vi "Get Optimal Fourier Order.vi"(8 "Error In":errorcluster, 9 "[b_k]":dbl[](array[numeric]), 11 "[a_k]":dbl[](array[numeric])) -> (0 "Error Out":errorcluster, 1 "Smoothed Power Spectrum":dbl[](array[numeric]), 3 "Optimal Fourier Order":i32)   [LabVIEW 2019]
uses:
  <vilib>/addons/_Advanced Signal Processing/NI_AdvSigProcTSA.lvlib
panel:
  out "Power Spectrum":dbl[](array[numeric])
  out "Graph":dbl[][](graph)
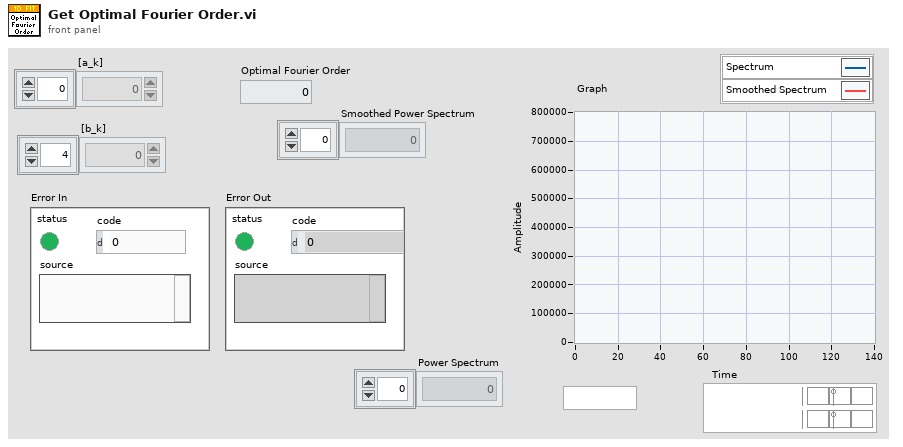
[diagram p1: front panel]
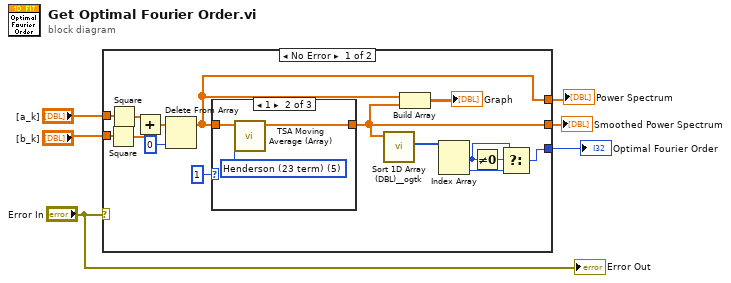
[diagram p0: block diagram]
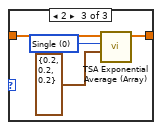
[diagram p3: hidden frame]
diagram:
  n1 = case shown="No Error" "Error In" {
    tunnel: "[a_k]" -> [w20 _]
    tunnel: "[b_k]" -> [w19 _]
    tunnel: [w12 _] -> w4
    tunnel: [w8 _] -> w3
    tunnel: [w10 _] -> w1
    frame No Error {
      n2 = Square(x=w19) -> (x^2=w18:dbl[])
      n3 = Square(x=w20) -> (x^2=w21:dbl[])
      n4 = Add(x=w21, y=w18) -> (x+y=w9:dbl[])
      n5 = Delete From Array(array=w9, index=0) -> (array with subset deleted=w8:dbl[])  [unwired: 1 in, 1 out]
      n6 = case shown="1" 1 {
        tunnel: w8 -> [w22 w25 w29]
        tunnel: [w22 w24 w28] -> w10
        frame 0, Default {
        }
        frame 1 {
          w23 = 5 items=["Spencer (15 term)"=1, "Henderson (7 term)"=2, "Henderson (9 term)"=3, "Henderson (13 term)"=4, "Henderson (23 term)"=5] ("method")
          n7 = call <vilib>:"TSA Moving Average (Array).vi"("method"=w23, "Xt"=w25) -> ("Xt out"=w24:dbl[])  [unwired: 8 in, 1 out]
        }
        frame 2 {
          w27 = u16 0 items=["Single", "Double", "Triple"] ("exponential type")
          n8 = call <vilib>:"TSA Exponential Average (Array).vi"("exponential factors"=cluster{"level":dbl, "trend":dbl, "season":dbl} {"level"=0.2, "trend"=0.2, "season"=0.2}, "exponential type"=w27, "Xt"=w29) -> ("Xt averaged"=w28:dbl[])  [unwired: 7 in, 1 out]
        }
      }
      n9 = call <userlib>:"Sort 1D Array (DBL)__ogtk.vi"("Array in"=w10) -> ("Sorted Pointers"=w16:i32[])  [unwired: 9 in, 1 out]
      n10 = Build Array(w8, w10) -> (→"Graph":dbl[][])
      n11 = Index Array(array=w16) -> (element #1=w14:i32, element #2=w13:i32)  [unwired: 2 in]
      n12 = Not Equal To 0?(x=w14) -> (x != 0?=w15:bool)
      n13 = Select(t=w14, s=w15, f=w13) -> (s? t:f=w12:i32)
    }
    frame Error {
    }
  }
  "Optimal Fourier Order" <- w4
  "Smoothed Power Spectrum" <- w1
  "Power Spectrum" <- w3
  "Error Out" <- "Error In"
